vi "Find Data Type.vi"(11 "String":string) -> (3 "Data Type":T1)   [LabVIEW 2022 SP3, in "hse-misc.lvlib"]
doc: "____\nHAMPEL SOFTWARE ENGINEERING v3.8.0 (2023-12-18 14:41)"
uses:
  hse-misc.lvlib
  <vilib>/Utility/Data Type/Type Definitions/Data Type.ctl
  <vilib>/regexp/Match Regular Expression.xnode
  <vilib>/Utility/Data Type/NI_Data Type.lvlib
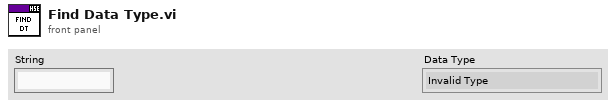
[diagram p1: front panel]
types:
  T1 = typedef "NI_Data Type.lvlib/Data Type.ctl" = enum8{"Invalid Type", "Void", "I8", "I16", "I32", "I64", "U8", "U16", "U32", "U64", "Single Float", "Double Float", "Extended Float", "Single Complex", "Double Complex", "Extended Complex", "Enum U8", "Enum U16", "Enum U32", "Enum U64", "Single Float With Unit", "Double Float With Unit", "Extended Float With Unit", "Single Complex with Unit", "Double Complex with Unit", "Extended Complex with Unit", "Boolean", "String", "Path", "Picture", "Tag", "Array", "Cluster", "Variant", "LV Variant", "Waveform", "Timestamp", "Digital Waveform", "Digital Data", "ExpressData", "Refnum", "External Data", "VI", "Poly VI", "LabVIEW Class Instance", "Fixed Point", "Set Collection", "Map Collection"}
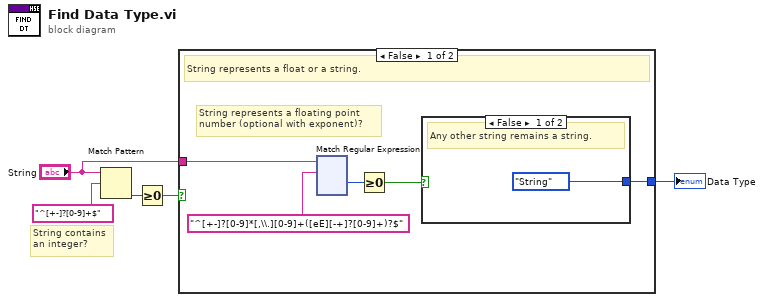
[diagram p0: block diagram]
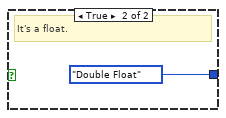
[diagram p2: hidden frame]
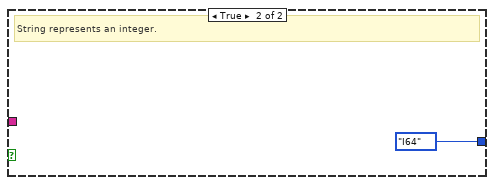
[diagram p3: hidden frame]
diagram:
  # "String contains\nan integer?"
  n1 = Match Pattern(string="String", regular expression="^[+-]?[0-9]+$") -> (offset past match=w2:i32)  [unwired: 1 in, 3 out]
  n2 = Greater Or Equal To 0?(x=w2) -> (x >= 0?=w1:bool)
  n3 = case shown="False" w1 {
    tunnel: [w6 Data_Type."I64" ("Type")] -> w5
    tunnel: "String" -> [w10 _]
    frame False {
      # "String represents a floating point \nnumber (optional with exponent)?"
      # "String represents a float or a string."
      n4 = xnode "Match Regular Expression"("input string"=w10, "regular expression"="^[+-]?[0-9]*[,\\.][0-9]+([eE][-+]?[0-9]+)?$") -> ("offset past match"=w8:i32)  [unwired: 4 in, 4 out]
      n5 = Greater Or Equal To 0?(x=w8) -> (x >= 0?=w7:bool)
      n6 = case shown="False" w7 {
        tunnel: [Data_Type."String" ("Type") Data_Type."Double Float" ("Type")] -> w6
        frame False {
          # "Any other string remains a string."
        }
        frame True {
          # "It's a float."
        }
      }
    }
    frame True {
      # "String represents an integer."
    }
  }
  "Data Type" <- w5
